vi "Open.vi"(0 "error handler in":refnum<class "TLB` Error Handler.lvclass">, 5 "error log path in":path, 11 "error in":errorcluster) -> (4 "error handler out":refnum<class "TLB` Error Handler.lvclass">, 15 "error out":errorcluster)   [LabVIEW 2015, in "TLB` Template.lvlib" / "TLB` Error Handler.lvclass"]
doc: "create and open resources used by the Error Handler.\n\n<B>Input Parameters</B>\n\n<B>error handler in</B> identifies your session. <B>Error Handler in</B> is obtained from the Open.vi of this class.\n\n<B>error log path in</B> destination of log file.\n\n<B>error in</B> describes error conditions that occur before this node runs. This input provides standard error in functionality.\n\n<B>Output Parameters</B>\n\n<B>error handler out</B> identifies your session. 'Error Handler out' is obtained from the Open.vi of this class.\n\n<B>error out</B> contains error information. This output provides standard error out functionality."
uses:
  TLB` Error Handler.lvclass
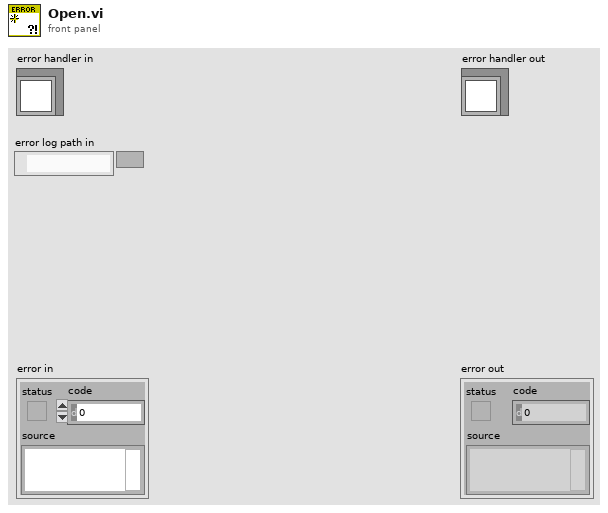
[diagram p1: front panel]
types:
  T1 = enum16{"open", "replace", "create", "open or create", "replace or create", "replace or create with confirmation"}
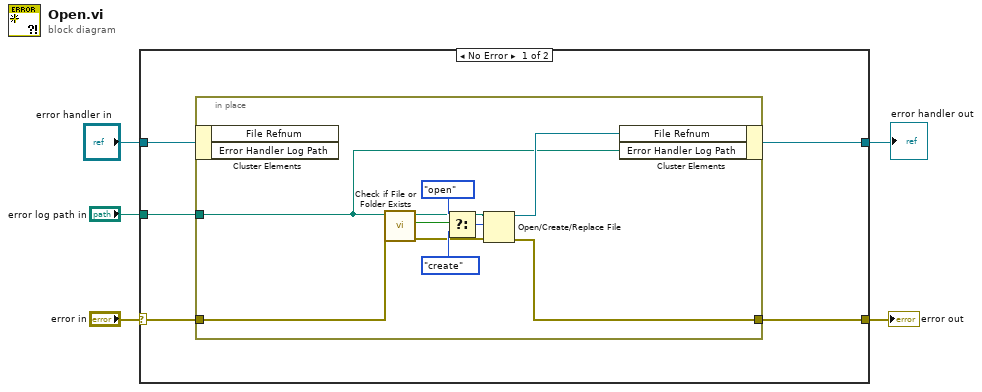
[diagram p0: block diagram]
diagram:
  n1 = case shown="No Error" "error in" {
    selector: "error in" -> [w9 w21]
    tunnel: "error handler in" -> [w10 w22]
    tunnel: [w8 w22] -> w3
    tunnel: [w7 w21] -> w2
    tunnel: "error log path in" -> [w6 _]
    frame No Error {
      n2 = in-place {
        in-place-border: w9 -> [w14]
        in-place-border: [w12] -> w7
        in-place-border: w6 -> [w11]
        n3 = in-place-cluster #1(w10) -> ()  [unwired: 2 out]
        n4 = call <vilib>:"Check if File or Folder Exists.vi"("error in (no error)"=w14, "path"=w11) -> ("error out"=w16:errorcluster, "file or folder exists?"=w15:bool, "dup path"=w17:path)  [unwired: 7 in]
        n5 = Select(t=T1."open" ("operation (0:open)"), s=w15, f=T1."create" ("operation (0:open)")) -> (s? t:f=w18:T1)
        n6 = Open/Create/Replace File(file path (use dialog)=w17, error in=w16, operation (0:open)=w18) -> (refnum out=w13:refnum<file>, error out=w12:errorcluster)  [unwired: 3 in, 1 out]
        n7 = in-place-cluster #1("File Refnum"=w13, "Error Handler Log Path"=w11) -> (w8:refnum<class "TLB` Error Handler.lvclass">)
      }
    }
    frame Error {
    }
  }
  "error out" <- w2
  "error handler out" <- w3
